vi "Door Closed Interlock Value Change.vi"(8 "error in (no error)":errorcluster, 10 "Door Closed Interlock":bool, 11 "Doors Opening in":refnum<class "Doors Opening.lvclass">) -> (0 "error out":errorcluster, 3 "Doors Opening out":refnum<class "Doors Opening.lvclass">)   [LabVIEW 2020, in "Door Controller.lvlib" / "Doors Opening.lvclass"]
uses:
  Doors Opening.lvclass
  C:/Users/Thomas.McQuillan/Desktop/Elevator Door Control/Door Controller/Door Controller/Door Controller.lvclass
  Application/Application/Interlock Names.ctl
  Door Controller/Door Controller.lvclass
  Application/Application.lvlib
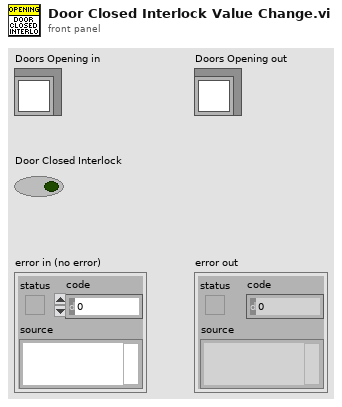
[diagram p1: front panel]
types:
  T1 = typedef "Application.lvlib/Interlock Names.ctl" = enum16{"Door Closed Interlock", "Door Open Interlock"}
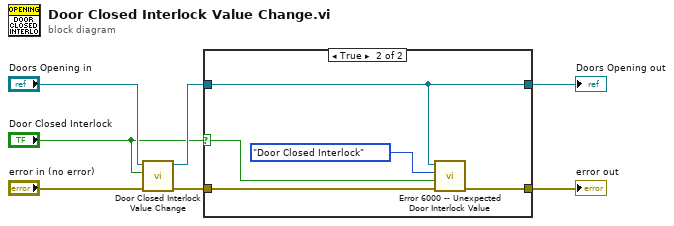
[diagram p0: block diagram]
diagram:
  n1 = call-parent "Door Closed Interlock Value Change.vi"("error in (no error)"="error in (no error)", "Door Closed Interlock"="Door Closed Interlock", "Door Controller in"="Doors Opening in") -> ("error out"=w3:errorcluster, "Door Controller out"=w5:refnum<class "Doors Opening.lvclass">)  [unwired: 7 in]
  n2 = case shown="True" "Door Closed Interlock" {
    selector: "Door Closed Interlock" -> [_ w10]
    tunnel: w5 -> [w9 w11]
    tunnel: [w9 w11] -> w4
    tunnel: w3 -> [w8 w13]
    tunnel: [w8 w12] -> w2
    frame False {
    }
    frame True {
      n3 = call "Error 6000 -- Unexpected Door Interlock Value.vi"("error in (no error)"=w13, "Interlock Value"=w10, "Interlock Name"=Interlock_Names."Door Closed Interlock", "Door Controller"=w11) -> ("error out"=w12:errorcluster)  [unwired: 7 in]
    }
  }
  "error out" <- w2
  "Doors Opening out" <- w4
